vi "Update Last Entry.vi"(8 "error in (no error)":errorcluster, 10 "New Entry":string[](array[string]) caption="New Entry (Table Row)", 11 "Cyclic Table in":refnum<class "Cyclic Table.lvclass">) -> (0 "error out":errorcluster, 3 "Cyclic Table out":refnum<class "Cyclic Table.lvclass">)   [LabVIEW 2024, in "Cyclic Table.lvclass"]
doc: "Update the text of the last entry (instead of making a new entry). This does not change the time of the entry."
uses:
  Cyclic Table.lvclass
  Cyclic Table.lvclass/Cyclic Table.ctl
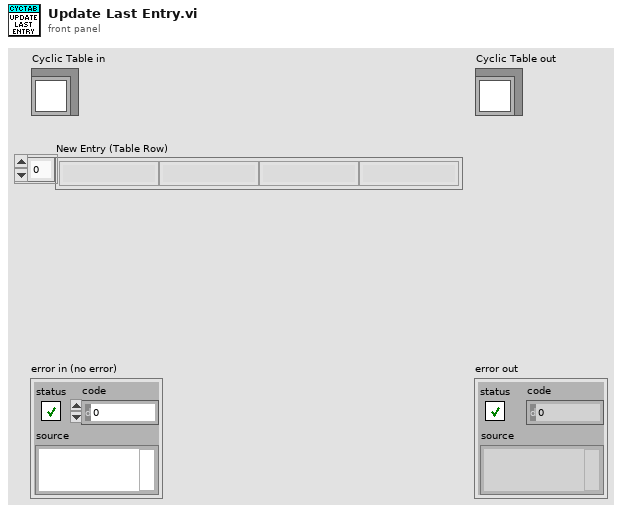
[diagram p1: front panel]
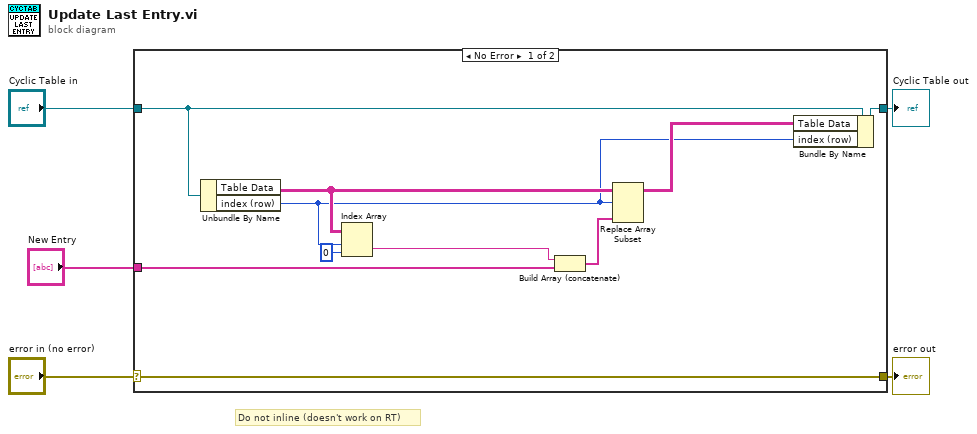
[diagram p0: block diagram]
diagram:
  # "Do not inline (doesn't work on RT)"
  n1 = case shown="No Error" "error in (no error)" {
    selector: "error in (no error)" -> [w15 w17]
    tunnel: [w15 w17] -> w4
    tunnel: [w12 w16] -> w2
    tunnel: "Cyclic Table in" -> [w13 w16]
    tunnel: "New Entry" -> [w11 _]
    frame No Error {
      n2 = Unbundle By Name(w13) -> ("Table Data"=w9:string[][], "index (row)"=w8:i32)
      n3 = Index Array(array=w9, index (row)=w8, index (col)=0 ("disabled index (col)")) -> (element=w6:string)
      n4 = Build Array (concatenate)(w6, w11) -> (w14:string[])
      n5 = Replace Array Subset(array=w9, new element=w14, index (row)=w8) -> (w10:string[][])  [unwired: 1 in]
      n6 = Bundle By Name(cluster=w13, "Table Data"=w10, "index (row)"=w8) -> (w12:refnum<class "Cyclic Table.lvclass">)
    }
    frame Error {
    }
  }
  "error out" <- w4
  "Cyclic Table out" <- w2
